vi "Enclose in Structure - Enclose Objects in Structure.vi"(7 "Top Level Diagram":refnum<vi>, 8 "error in":errorcluster, 10 "Structure Type":T1, 11 "Objects":refnum<vi>[](array[refnum])) -> (0 "error out":errorcluster, 3 "Structure":refnum<vi>)   [LabVIEW 2020]
uses:
  <vilib>/platform/TimedLoop/XDataNode/XDataNode.xnode
  <vilib>/Platform/TimedLoop/XDataNode/nitl_modes.ctl
  <vilib>/Platform/TimedLoop/XDataNode/XDNodeRunTimeDep.lvlib
  <vilib>/Platform/TimedLoop/XDataNode/wakeup.ctl
  <vilib>/Platform/TimedLoop/XDataNode/timing_clust.ctl
  <vilib>/Utility/traverseref.llb/TRef TravTarget.ctl
  Enclose in Structure - Structure Type.ctl
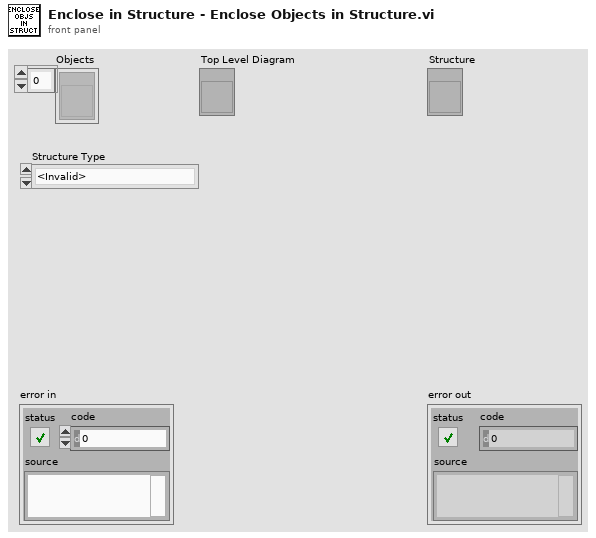
[diagram p1: front panel]
types:
  T1 = typedef "Enclose in Structure - Structure Type.ctl" = enum16{"<Invalid>", "For Loop", "While Loop", "Timed Loop", "Timed Sequence", "Case Structure", "Event Structure", "In Place Element Structure", "Flat Sequence", "Diagram Disable Structure", "Conditional Disable Structure", "Type Specialization Structure"}
  T2 = typedef "TRef TravTarget.ctl" = enum16{"FP", "BD", "Other"}
  T3 = typedef "XDNodeRunTimeDep.lvlib/timing_clust.ctl" = cluster{"Expected End [f-1]":u64, "Actual End [f-1]":u64, "Finished Late? [f-1]":bool, "Expected End [i-1]":u64, "Actual End [i-1]":u64, "Finished Late? [i-1]":bool, "Expected Start [i]":u64, "Actual Start [i]":u64, "Expected Start [f]":u64, "Actual Start [f]":u64, "Source Name":string, "Structure Name":string, "Period":i64, "Deadline":i64, "Offset":i64, "Start":i64, "Priority":i32, "Timeout":i32, "Mode":T4, "Wakeup Reason":T5, "Error":errorcluster, "Source Type":string, "Secondary Source Type":string, "Global End Time":u64, "Global Start Time":u64, "Frame Duration":u64, "Iteration Duration":u64, "Assigned CPU":i32, "I/O Scan Engine Mode":u32}
  T4 = typedef "XDNodeRunTimeDep.lvlib/nitl_modes.ctl" = enum32{"No Change", "Process missed periods, maintain original phase", "Discard missed periods, maintain original phase", "Process missed periods, ignore original phase", "Discard missed periods, ignore original phase"}
  T5 = typedef "XDNodeRunTimeDep.lvlib/wakeup.ctl" = enum32{"Normal", "Aborted", "Asynchronous wakeup", "Timing source error", "Timed loop error", "Timeout"}
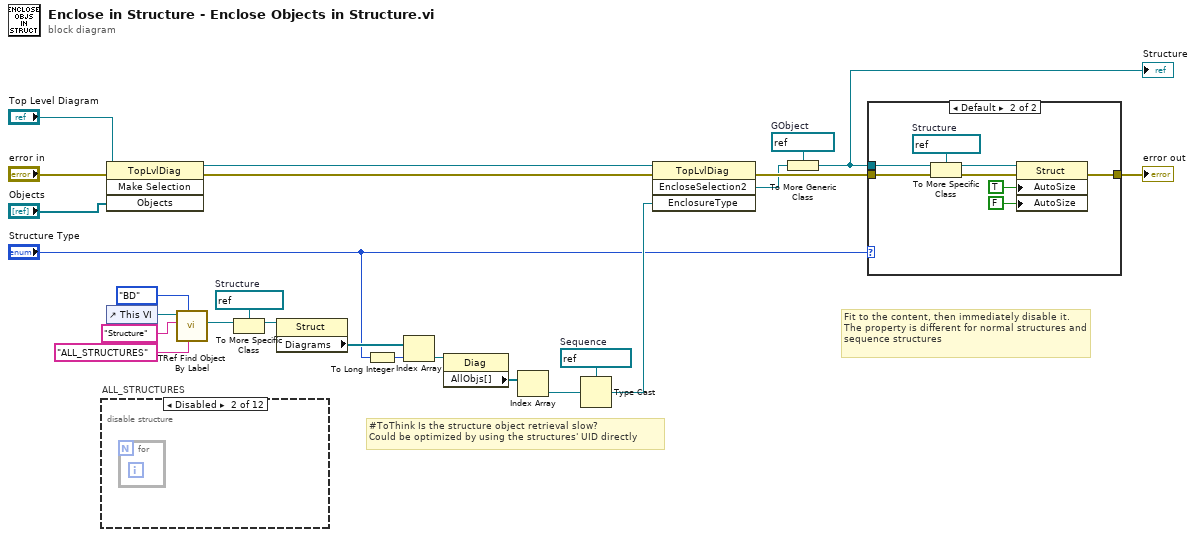
[diagram p0: block diagram]
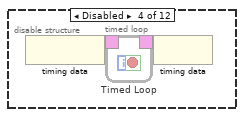
[diagram p4: hidden frame]
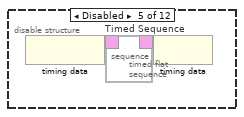
[diagram p5: hidden frame]
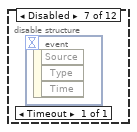
[diagram p8: hidden frame]
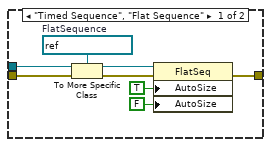
[diagram p16: hidden frame]
diagram:
  w3 = refnum<vi> refnum  # GObject
  w11 = refnum<vi> refnum  # Structure
  w24 = refnum<vi> refnum  # Sequence
  # "#ToThink Is the structure object retrieval slow?\nCould be optimized by using the structures' UID directly"
  # "Fit to the content, then immediately disable it.\nThe property is different for normal structures and sequence structures"
  n1 = disable-structure "ALL_STRUCTURES" shown="Disabled" {
    frame Enabled {
    }
    frame Disabled {
      n2 = for {
      }
    }
    frame Disabled {
      n3 = while {
        stop <- _ stop-if-true
      }
    }
    frame Disabled {
      n4 = node-c288() -> (w27:T3)
      n5 = timed-loop "Timed Loop" {
        timing: w27 -> [_]
        timing-out: [_] -> w26
        stop <- _ stop-if-true
      }
      n6 = node-c288(w26) -> ()
    }
    frame Disabled {
      n7 = node-c288() -> (w33:T3)
      n8 = timed-sequence "Timed Sequence" {
        timing: w33 -> [_]
        timing-out: [_] -> w32
        n9 = timed-flat-sequence {
        }
      }
      n10 = node-c288(w32) -> ()
    }
    frame Disabled {
      n11 = case shown="True" {
        selector: _ -> [_ _]
        frame False {
        }
        frame True {
        }
      }
    }
    frame Disabled {
      n12 = event shown="[0] Timeout" {
        selector: _ -> [_]
        dyn-events: _ -> [_]
        timeout: _ -> [_]
        event Timeout {
          n13 = event-data() -> ()  [unwired: 1 in, 3 out]
        }
      }
    }
    frame Disabled {
      n14 = in-place "In Place Element Structure" {
      }
    }
    frame Disabled {
      n15 = flat-sequence {
        frame #0 {
        }
      }
    }
    frame Disabled {
      n16 = disable-structure "Diagram Disable Structure" shown="Disabled" {
        frame Disabled {
        }
        frame Enabled {
        }
      }
    }
    frame Disabled {
      n17 = disable-structure "Conditional Disable Structure" shown="Default" {
        frame Enabled {
        }
      }
    }
    frame Disabled {
      n18 = disable-structure "Type Specialization Structure" shown="[0] Accepted" {
        frame Enabled {
        }
        frame Disabled {
        }
      }
    }
  }
  n19 = invoke class="TopLvlDiag" method="Make Selection"(reference="Top Level Diagram", error in="error in", "Objects"="Objects") -> (reference out=w22:refnum<vi>, error out=w21:errorcluster)  [unwired: 1 in, 2 out]
  n20 = control-ref of="This VI"() -> (w16:refnum<vi>)
  n21 = call <vilib>:"TRef Find Object By Label.vi"("Label"="ALL_STRUCTURES", "Traverse Target"=TRef_TravTarget."BD", "Class Name"="Structure", "VI Ref"=w16) -> ("Found Obj Ref"=w12:refnum<vi>)  [unwired: 4 in, 3 out]
  n22 = To More Specific Class(target class=w11, reference=w12) -> (specific class reference=w10:refnum<vi>)  [unwired: 1 in, 1 out]
  n23 = property class="Struct"(reference=w10) -> ("Diagrams"=w9:refnum<vi>[])  [unwired: 1 in, 2 out]
  n24 = To Long Integer(number="Structure Type") -> (32bit integer=w8:i32)
  n25 = Index Array(array=w9, index=w8) -> (element=w7:refnum<vi>)
  n26 = property class="Diag"(reference=w7) -> ("AllObjs[]"=w6:refnum<vi>[])  [unwired: 1 in, 2 out]
  n27 = Index Array(array=w6) -> (element=w5:refnum<vi>)  [unwired: 1 in]
  n28 = Type Cast(type=w24, x=w5) -> (*(type *) &x=w23:refnum<vi>)
  n29 = invoke class="TopLvlDiag" method="EncloseSelection2"(reference=w22, error in=w21, "EnclosureType"=w23) -> (error out=w25:errorcluster, "EncloseSelection2"=w2:refnum<vi>)  [unwired: 1 in, 2 out]
  n30 = To More Generic Class(target class=w3, reference=w2) -> (generic class reference=w1:refnum<vi>)
  "Structure" <- w1
  n31 = case shown="Default" "Structure Type" {
    tunnel: w25 -> [w45 w46]
    tunnel: w1 -> [w44 w48]
    tunnel: [w43 w53] -> w18
    frame "Timed Sequence", "Flat Sequence" {
      w42 = refnum<vi> refnum  # FlatSequence
      n32 = To More Specific Class(target class=w42, reference=w44, error in=w45) -> (specific class reference=w40:refnum<vi>, error out=w39:errorcluster)
      n33 = property class="FlatSeq"(reference=w40, error in=w39, "AutoSize"=TRUE ("AutoSize To Fit Contents?"), "AutoSize"=FALSE ("AutoSize To Fit Contents?")) -> (error out=w43:errorcluster)  [unwired: 1 out]
    }
    frame Default {
      w50 = refnum<vi> refnum  # Structure
      n34 = To More Specific Class(target class=w50, reference=w48, error in=w46) -> (specific class reference=w49:refnum<vi>, error out=w47:errorcluster)
      n35 = property class="Struct"(reference=w49, error in=w47, "AutoSize"=TRUE ("AutoSize To Fit Contents?"), "AutoSize"=FALSE ("AutoSize To Fit Contents?")) -> (error out=w53:errorcluster)  [unwired: 1 out]
    }
  }
  "error out" <- w18
